vi "Get ChanUsed_DC-Scope SP.vi"() -> (0 "ChanUsed":string)   [LabVIEW 2012]
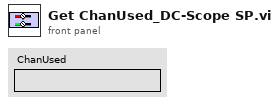
[diagram p1: front panel]
types:
  T1 = typedef "INI Initial Values_DStr-Scope SP.ctl" = cluster{"Active0":i32, "Acitive1":i32, "Channel":i32[], "ChanEnable":bool[], "ChanCpl":i32[], "OffsetVisible":bool[], "Offset":dbl[], "VoltInterval":i32[], "ProbAttenu":i32[], "Impedance":i32[], "BandWidth":i32[], "VertiPosi":dbl[], "Range":dbl[], "TimeInterval":i32, "Points":i32, "RefPosition":dbl, "Type":i32, "Source":i32, "TrigCpl":i32, "ExtCpl":i32, "Mode":i32, "Slope":i32, "Level":dbl, "Hyster":dbl, "WinMode":i32, "WinLow":dbl, "WinHigh":dbl, "Polarity":i32, "Event":i32, "Format":i32, "Line":i32, "DCRestore":bool, "RIS":bool, "Rate":dbl, "DigiSource":i32}
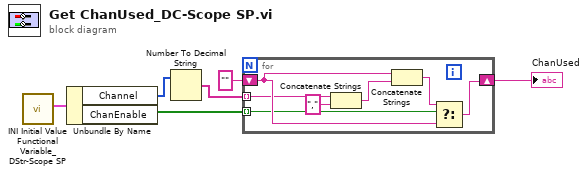
[diagram p0: block diagram]
diagram:
  n1 = call "INI Initial Value Functional Variable_DStr-Scope SP.vi"() -> ("Value out"=w4:T1)  [unwired: 10 in, 1 out]
  n2 = Unbundle By Name(w4) -> ("Channel"=w3:i32[], "ChanEnable"=w1:bool[])
  n3 = Number To Decimal String(number=w3) -> (decimal integer string=w2:string[])  [unwired: 1 in]
  n4 = for {
    shift-right: [w9] -> w6
    shift-left: "" -> [w10]
    tunnel: w2 -> [w8] mode=indexing
    tunnel: w1 -> [w7] mode=indexing
    n5 = Concatenate Strings(w8, "," ("string")) -> (w12:string)
    n6 = Concatenate Strings(w10, w12) -> (w11:string)
    n7 = Select(t=w11, s=w7, f=w10) -> (s? t:f=w9:string)
  }
  "ChanUsed" <- w6
